vi "6.2 - Convert to Neuron.vi"() -> (0 "6.7-Forebrain to OCU Neuron":T1 {"Current Waypoint"."X (waypoint)" format="%#_8g"; "Current Waypoint"."Y  (waypoint)" format="%#_8g"; "6.2-Where Am I? Sensor"."4.2.2- Current GPS Data"."Longitude (Decimal Degrees)" format="%#.6g"; "6.2-Where Am I? Sensor"."4.2.2- Current GPS Data"."Lattitude (Decimal Degrees)" format="%#.6g"})   [LabVIEW 2010]
uses:
  6.8-Forbrain to OCU neuron.ctl
  4-High Neurons/4.2-Where Sensor Typedef.ctl
  4-High Neurons/Current GPS Data.ctl
  3-Midbrain/3.2-Where/_typedefs/3.2.1-VectorNav Data.ctl
  6.1.11- Forbrain and midbrain Act neuron.ctl
  4-High Neurons/4.1-Midbrain Act Data.ctl
  6.4-How Reporting Typedef.ctl
  4-High Neurons/4.2/4.2.0 Kalman State.ctl
  5-Forebrain/5.0-Global.vi
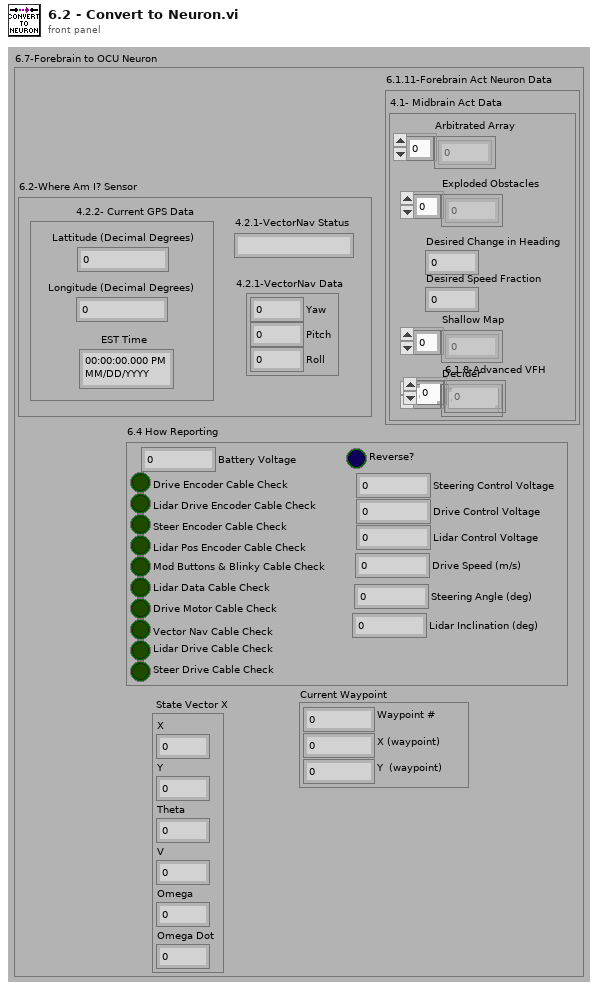
[diagram p1: front panel]
types:
  T1 = typedef "6.8-Forbrain to OCU neuron.ctl" = cluster{"6.2-Where Am I? Sensor":T2, "6.1.11-Forebrain Act Neuron Data":T5, "6.4 How Reporting":T7, "Current Waypoint":cluster{"Waypoint #":dbl, "X (waypoint)":ext, "Y  (waypoint)":ext}, " State Vector X":T8}
  T2 = typedef "4.2-Where Sensor Typedef.ctl" = cluster{"4.2.2- Current GPS Data":T3, "4.2.1-VectorNav Data":T4, "4.2.1-VectorNav Status":string}
  T3 = typedef "Current GPS Data.ctl" = cluster{"Lattitude (Decimal Degrees)":ext, "Longitude (Decimal Degrees)":ext, "EST Time":timestamp}
  T4 = typedef "3.2.1-VectorNav Data.ctl" = cluster{"Yaw":dbl, "Pitch":dbl, "Roll":dbl}
  T5 = typedef "6.1.11- Forbrain and midbrain Act neuron.ctl" = cluster{"4.1- Midbrain Act Data":T6, "6.1.8-Advanced VFH":dbl[]}
  T6 = typedef "4.1-Midbrain Act Data.ctl" = cluster{"Arbitrated Array":sgl[], "Exploded Obstacles":sgl[], "Desired Change in Heading":sgl, "Desired Speed Fraction":sgl, "Shallow Map":dbl[], "Decider":dbl[]}
  T7 = typedef "6.4-How Reporting Typedef.ctl" = cluster{"Drive Speed (m/s)":dbl, "Lidar Inclination (deg) ":dbl, "Steering Angle (deg)":dbl, "Battery Voltage":dbl, "Drive Encoder Cable Check":bool, "Lidar Drive Encoder Cable Check":bool, "Steer Encoder Cable Check":bool, "Lidar Pos Encoder Cable Check":bool, "Mod Buttons & Blinky Cable Check":bool, "Lidar Data Cable Check":bool, "Drive Motor Cable Check":bool, "Vector Nav Cable Check":bool, "Lidar Drive Cable Check":bool, "Steer Drive Cable Check":bool, "Reverse?":bool, "Steering Control Voltage":dbl, "Drive Control Voltage":dbl, "Lidar Control Voltage":dbl}
  T8 = typedef "4.2.0 Kalman State.ctl" = cluster{"X":dbl, "Y":dbl, "Theta":dbl, "V":dbl, "Omega":dbl, "Omega Dot":dbl}
  T9 = enum16{"Set Midbrain Act Data", "Set Forebrain Act Data", "Read Act Data"}
  T10 = typedef "MDF XY.ctl" = cluster{"Waypoint #":dbl, "X (waypoint)":ext, "Y  (waypoint)":ext}
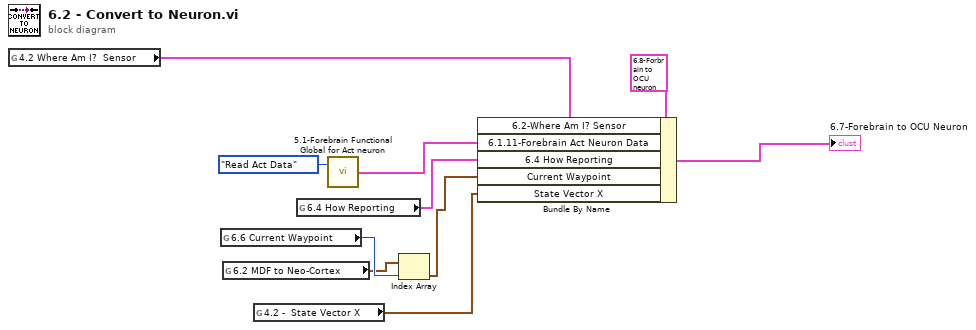
[diagram p0: block diagram]
diagram:
  n1 = global read "5.0-Global.vi" "4.2 Where Am I?  Sensor"() -> (w9:T2)
  n2 = global read "5.0-Global.vi" "6.6 Current Waypoint"() -> (w4:i32)
  n3 = global read "5.0-Global.vi" "6.2 MDF to Neo-Cortex"() -> (w3:T10[])
  n4 = global read "5.0-Global.vi" "4.2 -  State Vector X"() -> (w1:T8)
  n5 = global read "5.0-Global.vi" "6.4 How Reporting"() -> (w5:T7)
  n6 = call "5.1-Forebrain Functional Global for Act neuron.vi"("Command"=T9."Read Act Data") -> ("6.1.8-Forebrain Act Neuron Data"=w6:T5)  [unwired: 1 in]
  n7 = Index Array(array=w3, index=w4) -> (element=w2:T10)
  n8 = Bundle By Name(cluster=T1 {"6.2-Where Am I? Sensor"={"4.2.2- Current GPS Data"={"Lattitude (Decimal Degrees)"=0.0, "Longitude (Decimal Degrees)"=0.0, "EST Time"=timestamp(0 s since 1904-01-01)}, "4.2.1-VectorNav Data"={"Yaw"=0.0, "Pitch"=0.0, "Roll"=0.0}, "4.2.1-VectorNav Status"=""}, "6.1.11-Forebrain Act Neuron Data"={"4.1- Midbrain Act Data"={"Arbitrated Array"=[], "Exploded Obstacles"=[], "Desired Change in Heading"=0.0, "Desired Speed Fraction"=0.0, "Shallow Map"=[], "Decider"=[]}, "6.1.8-Advanced VFH"=[]}, "6.4 How Reporting"={"Drive Speed (m/s)"=0.0, "Lidar Inclination (deg) "=0.0, "Steering Angle (deg)"=0.0, "Battery Voltage"=0.0, "Drive Encoder Cable Check"=FALSE, "Lidar Drive Encoder Cable Check"=FALSE, "Steer Encoder Cable Check"=FALSE, "Lidar Pos Encoder Cable Check"=FALSE, "Mod Buttons & Blinky Cable Check"=FALSE, "Lidar Data Cable Check"=FALSE, "Drive Motor Cable Check"=FALSE, "Vector Nav Cable Check"=FALSE, "Lidar Drive Cable Check"=FALSE, "Steer Drive Cable Check"=FALSE, "Reverse?"=FALSE, "Steering Control Voltage"=0.0, "Drive Control Voltage"=0.0, "Lidar Control Voltage"=0.0}, "Current Waypoint"={"Waypoint #"=0.0, "X (waypoint)"=0.0, "Y  (waypoint)"=0.0}, " State Vector X"={"X"=0.0, "Y"=0.0, "Theta"=0.0, "V"=0.0, "Omega"=0.0, "Omega Dot"=0.0}} ("6.7-Forebrain to OCU Neuron"), "6.2-Where Am I? Sensor"=w9, "6.1.11-Forebrain Act Neuron Data"=w6, "6.4 How Reporting"=w5, "Current Waypoint"=w2, "State Vector X"=w1) -> (→"6.7-Forebrain to OCU Neuron":T1)
